vi "SERIAL_CalculateChecksum.vi"(4 "error in":errorcluster, 7 "Content":string) -> (0 "error out":errorcluster, 3 "Teminated Content":string)   [LabVIEW 2014]
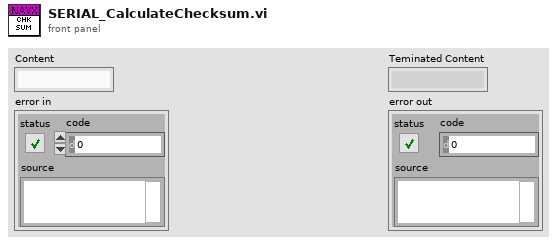
[diagram p1: front panel]
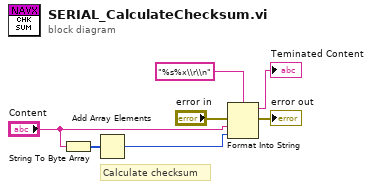
[diagram p0: block diagram]
diagram:
  # "Calculate checksum"
  n1 = String To Byte Array(string="Content") -> (unsigned byte array=w7:u8[])
  n2 = Add Array Elements(numeric array=w7) -> (sum=w5:u8)
  n3 = Format Into String(format string="%s%x\\r\\n" ("initial string"), error in="error in", "Content", w5) -> (resulting string=→"Teminated Content":string, error out=→"error out":errorcluster)  [unwired: 1 in]
